vi "Test Script Tree.vi"() -> ()   [LabVIEW 2020]
uses:
  typedefs/CC cluster Script.ctl
  typedefs/CC Script Step.ctl
  typedefs/CC enum Script Action.ctl
  CC Rd Wr Script Action.ctl
panel:
  out "Indent":i32[](array[numeric])
  out "All Tags":string[](array[string])
  in  "Multicolumn Listbox":i32(listbox)
  in  "index":i32
  out "Script List":string[](array[string])
  in  "Tree":string(tree)
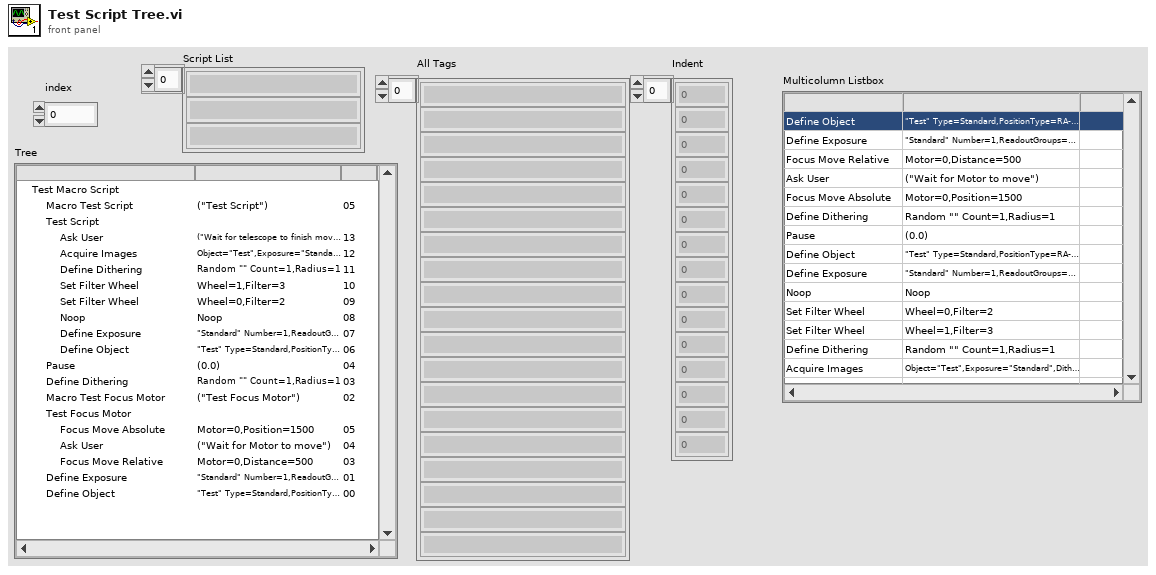
[diagram p1: front panel]
types:
  T1 = typedef "CC Rd Wr Script Action.ctl" = enum16{"Read", "Write", "List", "Delete"}
  T2 = typedef "CC cluster Script.ctl" = cluster{"Name":string, "Script":T3[]}
  T3 = typedef "CC Script Step.ctl" = cluster{"Action":T4, "Data":variant}
  T4 = typedef "CC enum Script Action.ctl" = enum16{"Noop", "Define Object", "Define Exposure", "Define Dithering", "Acquire Images", "Set Filter Wheel", "Focus Move Relative", "Focus Move Absolute", "Focus Set Home", "Macro", "Pause", "Ask User"}
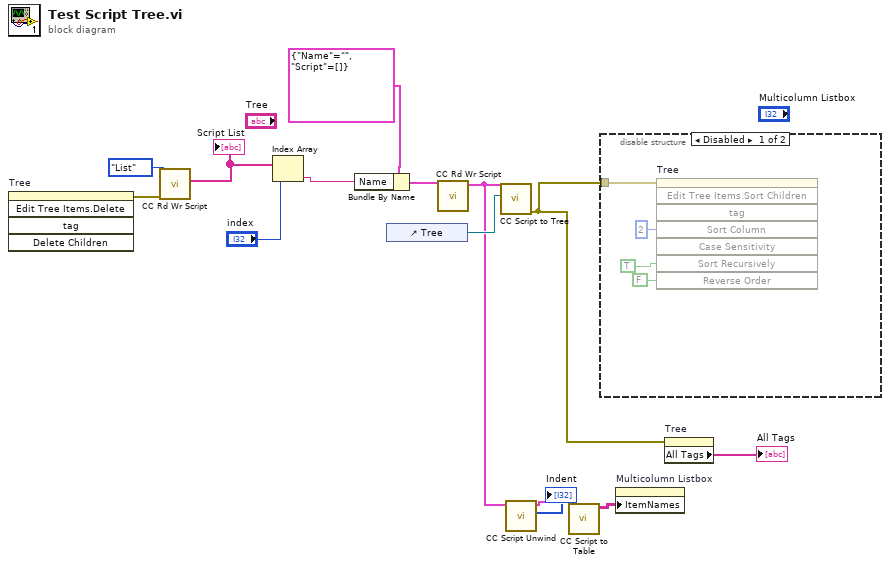
[diagram p0: block diagram]
diagram:
  n1 = invoke on="Tree" class="Tree (strict)" method="Edit Tree Items.Delete"() -> (error out=w8:errorcluster)  [unwired: 5 in, 4 out]
  n2 = call "CC Rd Wr Script.vi"("error in (no error)"=w8, "Action"=CC_Rd_Wr_Script_Action."List") -> ("Script List"=w14:string[])  [unwired: 5 in, 4 out]
  "Script List" <- w14
  n3 = Index Array(array=w14, index="index") -> (element=w12:string)
  n4 = Bundle By Name(cluster=T2 {"Name"="", "Script"=[]} ("Script"), "Name"=w12) -> (w11:T2)
  n5 = control-ref of="Tree"() -> (w10:refnum<vi>)
  n6 = call "CC Rd Wr Script.vi"("Script"=w11) -> ("Script"=w4:T2)  [unwired: 6 in, 4 out]
  n7 = call "CC Script to Tree.vi"("Tree ref"=w10, "Script"=w4) -> ("error out"=w6:errorcluster)  [unwired: 8 in, 1 out]
  n8 = call "CC Script Unwind.vi"("Script"=w4) -> ("Indent"=→"Indent":i32[], "Unwound Script"=w3:T3[])  [unwired: 8 in, 1 out]
  n9 = call "CC Script to Table.vi"("Script"=w3) -> ("table"=w7:string[][])  [unwired: 9 in, 1 out]
  n10 = disable-structure shown="Disabled" {
    disable-tunnel: w6 -> [w18 _]
    frame Disabled {
      n11 = invoke on="Tree" class="Tree (strict)" method="Edit Tree Items.Sort Children"(error in=w18, "Sort Column"=2, "Sort Recursively"=TRUE ("Reverse Order?"), "Reverse Order"=FALSE ("Reverse Order?")) -> ()  [unwired: 4 in, 8 out]
    }
    frame Enabled {
    }
  }
  n12 = property on="Multicolumn Listbox" class="MCListbox (strict)"("ItemNames"=w7) -> ()  [unwired: 2 in, 2 out]
  n13 = property on="Tree" class="Tree (strict)"(error in=w6) -> ("All Tags"=→"All Tags":string[])  [unwired: 1 in, 2 out]
